vi "Global 4 Gripper.vi"() -> ()   [LabVIEW 2022 SP3]
panel:
  in  "Numeric":i32
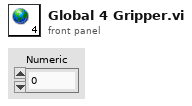
[diagram p1: front panel]
diagram:
